vi "Methods to Method Info.vi"(10 "Class":string, 11 "Methods from Node":T2(array[cluster])) -> (2 "Methods for Tree":T1(array[cluster]), 3 "Methods[]":T3(array[cluster]))   [LabVIEW 2023] (continued)
ID string"="22", "Class Name (unlocalized)"="WaveformGraph", "Class Name (localized)"="WaveformGraph"}, "Method Info"={"Unique ID string"="6343003", "Data name"="Export Data to Clipboard", "Short name (localized)"="Export Data to Clipboard", "Long name (localized)"="Export Data to Clipboard"}, "Method Flags"={"IsDeprecated"=FALSE, "IsPrivate"=FALSE, "IsScripting"=FALSE, "IsNotInRun-Time"=FALSE}, "Divider"=FALSE}, {"Class Info"={"Unique ID string"="24", "Parent ID string"="22", "Class Name (unlocalized)"="WaveformGraph", "Class Name (localized)"="WaveformGraph"}, "Method Info"={"Unique ID string"="6343004", "Data name"="Export Data to Excel", "Short name (localized)"="Export Data to Excel", "Long name (localized)"="Export Data to Excel"}, "Method Flags"={"IsDeprecated"=FALSE, "IsPrivate"=FALSE, "IsScripting"=FALSE, "IsNotInRun-Time"=FALSE}, "Divider"=FALSE}, {"Class Info"={"Unique ID string"="24", "Parent ID string"="22", "Class Name (unlocalized)"="WaveformGraph", "Class Name (localized)"="WaveformGraph"}, "Method Info"={"Unique ID string"="6343005", "Data name"="Export Data to DIAdem", "Short name (localized)"="Export Data to DIAdem", "Long name (localized)"="Export Data to DIAdem"}, "Method Flags"={"IsDeprecated"=FALSE, "IsPrivate"=FALSE, "IsScripting"=FALSE, "IsNotInRun-Time"=FALSE}, "Divider"=FALSE}, {"Class Info"={"Unique ID string"="24", "Parent ID string"="22", "Class Name (unlocalized)"="WaveformGraph", "Class Name (localized)"="WaveformGraph"}, "Method Info"={"Unique ID string"="6343006", "Data name"="Export Plot Data To Clipboard", "Short name (localized)"="Export Plot Data To Clipboard", "Long name (localized)"="Export Plot Data To Clipboard"}, "Method Flags"={"IsDeprecated"=FALSE, "IsPrivate"=FALSE, "IsScripting"=FALSE, "IsNotInRun-Time"=FALSE}, "Divider"=FALSE}, {"Class Info"={"Unique ID string"="24", "Parent ID string"="22", "Class Name (unlocalized)"="WaveformGraph", "Class Name (localized)"="WaveformGraph"}, "Method Info"={"Unique ID string"="6343007", "Data name"="Export Plot Data To Excel", "Short name (localized)"="Export Plot Data To Excel", "Long name (localized)"="Export Plot Data To Excel"}, "Method Flags"={"IsDeprecated"=FALSE, "IsPrivate"=FALSE, "IsScripting"=FALSE, "IsNotInRun-Time"=FALSE}, "Divider"=FALSE}, {"Class Info"={"Unique ID string"="24", "Parent ID string"="22", "Class Name (unlocalized)"="WaveformGraph", "Class Name (localized)"="WaveformGraph"}, "Method Info"={"Unique ID string"="6343008", "Data name"="Export Plot Data To DIAdem", "Short name (localized)"="Export Plot Data To DIAdem", "Long name (localized)"="Export Plot Data To DIAdem"}, "Method Flags"={"IsDeprecated"=FALSE, "IsPrivate"=FALSE, "IsScripting"=FALSE, "IsNotInRun-Time"=FALSE}, "Divider"=FALSE}, {"Class Info"={"Unique ID string"="25", "Parent ID string"="22", "Class Name (unlocalized)"="IntensityChart", "Class Name (localized)"="IntensityChart"}, "Method Info"={"Unique ID string"="6343c00", "Data name"="Export Data to Clipboard", "Short name (localized)"="Export Data to Clipboard", "Long name (localized)"="Export Data to Clipboard"}, "Method Flags"={"IsDeprecated"=FALSE, "IsPrivate"=FALSE, "IsScripting"=FALSE, "IsNotInRun-Time"=FALSE}, "Divider"=FALSE}, {"Class Info"={"Unique ID string"="25", "Parent ID string"="22", "Class Name (unlocalized)"="IntensityChart", "Class Name (localized)"="IntensityChart"}, "Method Info"={"Unique ID string"="6343c01", "Data name"="Export Data to Excel", "Short name (localized)"="Export Data to Excel", "Long name (localized)"="Export Data to Excel"}, "Method Flags"={"IsDeprecated"=FALSE, "IsPrivate"=FALSE, "IsScripting"=FALSE, "IsNotInRun-Time"=FALSE}, "Divider"=FALSE}, {"Class Info"={"Unique ID string"="26", "Parent ID string"="22", "Class Name (unlocalized)"="IntensityGraph", "Class Name (localized)"="IntensityGraph"}, "Method Info"={"Unique ID string"="6344800", "Data name"="Export Data to Clipboard", "Short name (localized)"="Export Data to Clipboard", "Long name (localized)"="Export Data to Clipboard"}, "Method Flags"={"IsDeprecated"=FALSE, "IsPrivate"=FALSE, "IsScripting"=FALSE, "IsNotInRun-Time"=FALSE}, "Divider"=FALSE}, {"Class Info"={"Unique ID string"="26", "Parent ID string"="22", "Class Name (unlocalized)"="IntensityGraph", "Class Name (localized)"="IntensityGraph"}, "Method Info"={"Unique ID string"="6344801", "Data name"="Export Data to Excel", "Short name (localized)"="Export Data to Excel", "Long name (localized)"="Export Data to Excel"}, "Method Flags"={"IsDeprecated"=FALSE, "IsPrivate"=FALSE, "IsScripting"=FALSE, "IsNotInRun-Time"=FALSE}, "Divider"=FALSE}, {"Class Info"={"Unique ID string"="27", "Parent ID string"="6", "Class Name (unlocalized)"="String", "Class Name (localized)"="String"}, "Method Info"={"Unique ID string"="6345400", "Data name"="Size to Text", "Short name (localized)"="Size to Text", "Long name (localized)"="Size to Text"}, "Method Flags"={"IsDeprecated"=FALSE, "IsPrivate"=FALSE, "IsScripting"=FALSE, "IsNotInRun-Time"=FALSE}, "Divider"=FALSE}, {"Class Info"={"Unique ID string"="27", "Parent ID string"="6", "Class Name (unlocalized)"="String", "Class Name (localized)"="String"}, "Method Info"={"Unique ID string"="6345401", "Data name"="Get Nth Line", "Short name (localized)"="Get Nth Line", "Long name (localized)"="Get Nth Line"}, "Method Flags"={"IsDeprecated"=FALSE, "IsPrivate"=FALSE, "IsScripting"=FALSE, "IsNotInRun-Time"=FALSE}, "Divider"=FALSE}, {"Class Info"={"Unique ID string"="27", "Parent ID string"="6", "Class Name (unlocalized)"="String", "Class Name (localized)"="String"}, "Method Info"={"Unique ID string"="6345402", "Data name"="ByteOffFromPt", "Short name (localized)"="ByteOffFromPt", "Long name (localized)"="Byte Offset from Point"}, "Method Flags"={"IsDeprecated"=FALSE, "IsPrivate"=FALSE, "IsScripting"=FALSE, "IsNotInRun-Time"=FALSE}, "Divider"=FALSE}, {"Class Info"={"Unique ID string"="27", "Parent ID string"="6", "Class Name (unlocalized)"="String", "Class Name (localized)"="String"}, "Method Info"={"Unique ID string"="6345403", "Data name"="Append String", "Short name (localized)"="Append String", "Long name (localized)"="Append String"}, "Method Flags"={"IsDeprecated"=FALSE, "IsPrivate"=FALSE, "IsScripting"=FALSE, "IsNotInRun-Time"=FALSE}, "Divider"=FALSE}, {"Class Info"={"Unique ID string"="30", "Parent ID string"="6", "Class Name (unlocalized)"="Cluster", "Class Name (localized)"="Cluster"}, "Method Info"={"Unique ID string"="6347800", "Data name"="Set Cluster Order", "Short name (localized)"="Set Cluster Order", "Long name (localized)"="Set Cluster Order"}, "Method Flags"={"IsDeprecated"=FALSE, "IsPrivate"=FALSE, "IsScripting"=TRUE, "IsNotInRun-Time"=FALSE}, "Divider"=FALSE}, {"Class Info"={"Unique ID string"="31", "Parent ID string"="36", "Class Name (unlocalized)"="Panel", "Class Name (localized)"="Panel"}, "Method Info"={"Unique ID string"="6348400", "Data name"="Set Panel Order", "Short name (localized)"="Set Panel Order", "Long name (localized)"="Set Panel Order"}, "Method Flags"={"IsDeprecated"=FALSE, "IsPrivate"=FALSE, "IsScripting"=TRUE, "IsNotInRun-Time"=FALSE}, "Divider"=FALSE}, {"Class Info"={"Unique ID string"="31", "Parent ID string"="36", "Class Name (unlocalized)"="Panel", "Class Name (localized)"="Panel"}, "Method Info"={"Unique ID string"="6348402", "Data name"="Clear Selection", "Short name (localized)"="Clear Selection", "Long name (localized)"="Clear Selection"}, "Method Flags"={"IsDeprecated"=FALSE, "IsPrivate"=FALSE, "IsScripting"=TRUE, "IsNotInRun-Time"=TRUE}, "Divider"=FALSE}, {"Class Info"={"Unique ID string"="31", "Parent ID string"="36", "Class Name (unlocalized)"="Panel", "Class Name (localized)"="Panel"}, "Method Info"={"Unique ID string"="6348403", "Data name"="Make Selection", "Short name (localized)"="Make Selection", "Long name (localized)"="Make Selection"}, "Method Flags"={"IsDeprecated"=FALSE, "IsPrivate"=FALSE, "IsScripting"=TRUE, "IsNotInRun-Time"=TRUE}, "Divider"=FALSE}, {"Class Info"={"Unique ID string"="31", "Parent ID string"="36", "Class Name (unlocalized)"="Panel", "Class Name (localized)"="Panel"}, "Method Info"={"Unique ID string"="6348404", "Data name"="Select All", "Short name (localized)"="Select All", "Long name (localized)"="Select All"}, "Method Flags"={"IsDeprecated"=FALSE, "IsPrivate"=FALSE, "IsScripting"=TRUE, "IsNotInRun-Time"=TRUE}, "Divider"=FALSE}, {"Class Info"={"Unique ID string"="31", "Parent ID string"="36", "Class Name (unlocalized)"="Panel", "Class Name (localized)"="Panel"}, "Method Info"={"Unique ID string"="6348405", "Data name"="Copy Selection", "Short name (localized)"="Copy Selection", "Long name (localized)"="Copy Selection"}, "Method Flags"={"IsDeprecated"=FALSE, "IsPrivate"=FALSE, "IsScripting"=TRUE, "IsNotInRun-Time"=TRUE}, "Divider"=FALSE}, {"Class Info"={"Unique ID string"="31", "Parent ID string"="36", "Class Name (unlocalized)"="Panel", "Class Name (localized)"="Panel"}, "Method Info"={"Unique ID string"="634840b", "Data name"="MoveSelectionToFront", "Short name (localized)"="MoveSelectionToFront", "Long name (localized)"="Move Selection To Front"}, "Method Flags"={"IsDeprecated"=FALSE, "IsPrivate"=FALSE, "IsScripting"=TRUE, "IsNotInRun-Time"=TRUE}, "Divider"=FALSE}, {"Class Info"={"Unique ID string"="31", "Parent ID string"="36", "Class Name (unlocalized)"="Panel", "Class Name (localized)"="Panel"}, "Method Info"={"Unique ID string"="634840c", "Data name"="MoveSelectionToBack", "Short name (localized)"="MoveSelectionToBack", "Long name (localized)"="Move Selection To Back"}, "Method Flags"={"IsDeprecated"=FALSE, "IsPrivate"=FALSE, "IsScripting"=TRUE, "IsNotInRun-Time"=TRUE}, "Divider"=FALSE}, {"Class Info"={"Unique ID string"="31", "Parent ID string"="36", "Class Name (unlocalized)"="Panel", "Class Name (localized)"="Panel"}, "Method Info"={"Unique ID string"="634840d", "Data name"="MoveSelectionForward", "Short name (localized)"="MoveSelectionForward", "Long name (localized)"="Move Selection Forward"}, "Method Flags"={"IsDeprecated"=FALSE, "IsPrivate"=FALSE, "IsScripting"=TRUE, "IsNotInRun-Time"=TRUE}, "Divider"=FALSE}, {"Class Info"={"Unique ID string"="31", "Parent ID string"="36", "Class Name (unlocalized)"="Panel", "Class Name (localized)"="Panel"}, "Method Info"={"Unique ID string"="634840e", "Data name"="MoveSelectionBackward", "Short name (localized)"="MoveSelectionBackward", "Long name (localized)"="Move Selection Backward"}, "Method Flags"={"IsDeprecated"=FALSE, "IsPrivate"=FALSE, "IsScripting"=TRUE, "IsNotInRun-Time"=TRUE}, "Divider"=FALSE}, {"Class Info"={"Unique ID string"="31", "Parent ID string"="36", "Class Name (unlocalized)"="Panel", "Class Name (localized)"="Panel"}, "Method Info"={"Unique ID string"="634840f", "Data name"="CvtPanelToScreenCoords", "Short name (localized)"="CvtPanelToScreenCoords", "Long name (localized)"="Convert Panel To Screen Coordinates"}, "Method Flags"={"IsDeprecated"=FALSE, "IsPrivate"=FALSE, "IsScripting"=FALSE, "IsNotInRun-Time"=FALSE}, "Divider"=FALSE}, {"Class Info"={"Unique ID string"="31", "Parent ID string"="36", "Class Name (unlocalized)"="Panel", "Class Name (localized)"="Panel"}, "Method Info"={"Unique ID string"="6348410", "Data name"="CvtScreenToPanelCoords", "Short name (localized)"="CvtScreenToPanelCoords", "Long name (localized)"="Convert Screen To Panel Coordinates"}, "Method Flags"={"IsDeprecated"=FALSE, "IsPrivate"=FALSE, "IsScripting"=FALSE, "IsNotInRun-Time"=FALSE}, "Divider"=FALSE}, {"Class Info"={"Unique ID string"="31", "Parent ID string"="36", "Class Name (unlocalized)"="Panel", "Class Name (localized)"="Panel"}, "Method Info"={"Unique ID string"="6348411", "Data name"="DistributeSelection", "Short name (localized)"="DistributeSelection", "Long name (localized)"="Distribute Selection"}, "Method Flags"={"IsDeprecated"=FALSE, "IsPrivate"=FALSE, "IsScripting"=TRUE, "IsNotInRun-Time"=TRUE}, "Divider"=FALSE}, {"Class Info"={"Unique ID string"="31", "Parent ID string"="36", "Class Name (unlocalized)"="Panel", "Class Name (localized)"="Panel"}, "Method Info"={"Unique ID string"="6348412", "Data name"="AlignSelection", "Short name (localized)"="AlignSelection", "Long name (localized)"="Align Selection"}, "Method Flags"={"IsDeprecated"=FALSE, "IsPrivate"=FALSE, "IsScripting"=TRUE, "IsNotInRun-Time"=TRUE}, "Divider"=FALSE}, {"Class Info"={"Unique ID string"="33", "Parent ID string"="17", "Class Name (unlocalized)"="NumericWithScale", "Class Name (localized)"="NumericWithScale"}, "Method Info"={"Unique ID string"="633f400", "Data name"="Add Slider", "Short name (localized)"="Add Slider", "Long name (localized)"="Add Slider"}, "Method Flags"={"IsDeprecated"=FALSE, "IsPrivate"=FALSE, "IsScripting"=TRUE, "IsNotInRun-Time"=TRUE}, "Divider"=FALSE}, {"Class Info"={"Unique ID string"="33", "Parent ID string"="17", "Class Name (unlocalized)"="NumericWithScale", "Class Name (localized)"="NumericWithScale"}, "Method Info"={"Unique ID string"="633f401", "Data name"="Delete Slider", "Short name (localized)"="Delete Slider", "Long name (localized)"="Delete Slider"}, "Method Flags"={"IsDeprecated"=FALSE, "IsPrivate"=FALSE, "IsScripting"=TRUE, "IsNotInRun-Time"=TRUE}, "Divider"=FALSE}, {"Class Info"={"Unique ID string"="36", "Parent ID string"="3", "Class Name (unlocalized)"="GObject", "Class Name (localized)"="GObject"}, "Method Info"={"Unique ID string"="632a400", "Data name"="Move", "Short name (localized)"="Move", "Long name (localized)"="Move"}, "Method Flags"={"IsDeprecated"=FALSE, "IsPrivate"=FALSE, "IsScripting"=TRUE, "IsNotInRun-Time"=TRUE}, "Divider"=FALSE}, {"Class Info"={"Unique ID string"="36", "Parent ID string"="3", "Class Name (unlocalized)"="GObject", "Class Name (localized)"="GObject"}, "Method Info"={"Unique ID string"="632a401", "Data name"="ObjHighlight", "Short name (localized)"="ObjHighlight", "Long name (localized)"="Object Highlight"}, "Method Flags"={"IsDeprecated"=FALSE, "IsPrivate"=FALSE, "IsScripting"=FALSE, "IsNotInRun-Time"=FALSE}, "Divider"=FALSE}, {"Class Info"={"Unique ID string"="36", "Parent ID string"="3", "Class Name (unlocalized)"="GObject", "Class Name (localized)"="GObject"}, "Method Info"={"Unique ID string"="632a402", "Data name"="Replace", "Short name (localized)"="Replace", "Long name (localized)"="Replace"}, "Method Flags"={"IsDeprecated"=FALSE, "IsPrivate"=FALSE, "IsScripting"=TRUE, "IsNotInRun-Time"=TRUE}, "Divider"=FALSE}, {"Class Info"={"Unique ID string"="36", "Parent ID string"="3", "Class Name (unlocalized)"="GObject", "Class Name (localized)"="GObject"}, "Method Info"={"Unique ID string"="632a403", "Data name"="Replace No Attrib", "Short name (localized)"="Replace No Attrib", "Long name (localized)"="Replace No Attributes"}, "Method Flags"={"IsDeprecated"=FALSE, "IsPrivate"=FALSE, "IsScripting"=TRUE, "IsNotInRun-Time"=TRUE}, "Divider"=FALSE}, {"Class Info"={"Unique ID string"="36", "Parent ID string"="3", "Class Name (unlocalized)"="GObject", "Class Name (localized)"="GObject"}, "Method Info"={"Unique ID string"="632a404", "Data name"="Launch Config", "Short name (localized)"="Launch Config", "Long name (localized)"="Launch Config Page"}, "Method Flags"={"IsDeprecated"=FALSE, "IsPrivate"=TRUE, "IsScripting"=TRUE, "IsNotInRun-Time"=TRUE}, "Divider"=FALSE}, {"Class Info"={"Unique ID string"="36", "Parent ID string"="3", "Class Name (unlocalized)"="GObject", "Class Name (localized)"="GObject"}, "Method Info"={"Unique ID string"="632a405", "Data name"="Invalidate", "Short name (localized)"="Invalidate", "Long name (localized)"="Invalidate"}, "Method Flags"={"IsDeprecated"=FALSE, "IsPrivate"=TRUE, "IsScripting"=TRUE, "IsNotInRun-Time"=FALSE}, "Divider"=FALSE}, {"Class Info"={"Unique ID string"="36", "Parent ID string"="3", "Class Name (unlocalized)"="GObject", "Class Name (localized)"="GObject"}, "Method Info"={"Unique ID string"="632a406", "Data name"="ReplacePreferringStubDDOOnFP", "Short name (localized)"="ReplacePreferringStubDDOOnFP", "Long name (localized)"="Replace Preferring Stub DDO OnFP"}, "Method Flags"={"IsDeprecated"=FALSE, "IsPrivate"=TRUE, "IsScripting"=TRUE, "IsNotInRun-Time"=TRUE}, "Divider"=FALSE}, {"Class Info"={"Unique ID string"="36", "Parent ID string"="3", "Class Name (unlocalized)"="GObject", "Class Name (localized)"="GObject"}, "Method Info"={"Unique ID string"="632a407", "Data name"="GetObjHelp", "Short name (localized)"="GetObjHelp", "Long name (localized)"="Get Help Info"}, "Method Flags"={"IsDeprecated"=FALSE, "IsPrivate"=FALSE, "IsScripting"=TRUE, "IsNotInRun-Time"=FALSE}, "Divider"=FALSE}, {"Class Info"={"Unique ID string"="46", "Parent ID string"="6", "Class Name (unlocalized)"="MulticolumnListbox", "Class Name (localized)"="MulticolumnListbox"}, "Method Info"={"Unique ID string"="18d99400", "Data name"="Get DblClk Row", "Short name (localized)"="Get DblClk Row", "Long name (localized)"="Get Double-Clicked Row"}, "Method Flags"={"IsDeprecated"=FALSE, "IsPrivate"=FALSE, "IsScripting"=FALSE, "IsNotInRun-Time"=FALSE}, "Divider"=FALSE}, {"Class Info"={"Unique ID string"="46", "Parent ID string"="6", "Class Name (unlocalized)"="MulticolumnListbox", "Class Name (localized)"="MulticolumnListbox"}, "Method Info"={"Unique ID string"="18d99401", "Data name"="Get Clicked Col Hdr", "Short name (localized)"="Get Clicked Col Hdr", "Long name (localized)"="Get Clicked Column Header"}, "Method Flags"={"IsDeprecated"=FALSE, "IsPrivate"=FALSE, "IsScripting"=FALSE, "IsNotInRun-Time"=FALSE}, "Divider"=FALSE}, {"Class Info"={"Unique ID string"="46", "Parent ID string"="6", "Class Name (unlocalized)"="MulticolumnListbox", "Class Name (localized)"="MulticolumnListbox"}, "Method Info"={"Unique ID string"="18d99402", "Data name"="Point To Row Column", "Short name (localized)"="Point To Row Column", "Long name (localized)"="Point to Row Column"}, "Method Flags"={"IsDeprecated"=FALSE, "IsPrivate"=FALSE, "IsScripting"=FALSE, "IsNotInRun-Time"=FALSE}, "Divider"=FALSE}, {"Class Info"={"Unique ID string"="46", "Parent ID string"="6", "Class Name (unlocalized)"="MulticolumnListbox", "Class Name (localized)"="MulticolumnListbox"}, "Method Info"={"Unique ID string"="18d99403", "Data name"="Custom Item Symbols.Get Symbol", "Short name (localized)"="Custom Item Symbols.Get Symbol", "Long name (localized)"="Custom Item Symbols:Get Symbol"}, "Method Flags"={"IsDeprecated"=FALSE, "IsPrivate"=FALSE, "IsScripting"=FALSE, "IsNotInRun-Time"=FALSE}, "Divider"=FALSE}, {"Class Info"={"Unique ID string"="46", "Parent ID string"="6", "Class Name (unlocalized)"="MulticolumnListbox", "Class Name (localized)"="MulticolumnListbox"}, "Method Info"={"Unique ID string"="18d99404", "Data name"="Custom Item Symbols.Get Symbol Array", "Short name (localized)"="Custom Item Symbols.Get Symbol Array", "Long name (localized)"="Custom Item Symbols:Get Symbol Array"}, "Method Flags"={"IsDeprecated"=FALSE, "IsPrivate"=FALSE, "IsScripting"=FALSE, "IsNotInRun-Time"=FALSE}, "Divider"=FALSE}, {"Class Info"={"Unique ID string"="46", "Parent ID string"="6", "Class Name (unlocalized)"="MulticolumnListbox", "Class Name (localized)"="MulticolumnListbox"}, "Method Info"={"Unique ID string"="18d99405", "Data name"="Custom Item Symbols.Set Symbol", "Short name (localized)"="Custom Item Symbols.Set Symbol", "Long name (localized)"="Custom Item Symbols:Set To Custom Symbol"}, "Method Flags"={"IsDeprecated"=FALSE, "IsPrivate"=FALSE, "IsScripting"=FALSE, "IsNotInRun-Time"=FALSE}, "Divider"=FALSE}, {"Class Info"={"Unique ID string"="46", "Parent ID string"="6", "Class Name (unlocalized)"="MulticolumnListbox", "Class Name (localized)"="MulticolumnListbox"}, "Method Info"={"Unique ID string"="18d99406", "Data name"="Custom Item Symbols.Set Symbol Array", "Short name (localized)"="Custom Item Symbols.Set Symbol Array", "Long name (localized)"="Custom Item Symbols:Set To Custom Symbol Array"}, "Method Flags"={"IsDeprecated"=FALSE, "IsPrivate"=FALSE, "IsScripting"=FALSE, "IsNotInRun-Time"=FALSE}, "Divider"=FALSE}, {"Class Info"={"Unique ID string"="46", "Parent ID string"="6", "Class Name (unlocalized)"="MulticolumnListbox", "Class Name (localized)"="MulticolumnListbox"}, "Method Info"={"Unique ID string"="18d99407", "Data name"="Custom Item Symbols.Revert Symbol", "Short name (localized)"="Custom Item Symbols.Revert Symbol", "Long name (localized)"="Custom Item Symbols:Revert To Built In Symbol"}, "Method Flags"={"IsDeprecated"=FALSE, "IsPrivate"=FALSE, "IsScripting"=FALSE, "IsNotInRun-Time"=FALSE}, "Divider"=FALSE}, {"Class Info"={"Unique ID string"="46", "Parent ID string"="6", "Class Name (unlocalized)"="MulticolumnListbox", "Class Name (localized)"="MulticolumnListbox"}, "Method Info"={"Unique ID string"="18d99408", "Data name"="Custom Item Symbols.Revert Symbols", "Short name (localized)"="Custom Item Symbols.Revert Symbols", "Long name (localized)"="Custom Item Symbols:Revert All To Built In Symbols"}, "Method Flags"={"IsDeprecated"=FALSE, "IsPrivate"=FALSE, "IsScripting"=FALSE, "IsNotInRun-Time"=FALSE}, "Divider"=FALSE}, {"Class Info"={"Unique ID string"="50", "Parent ID string"="28", "Class Name (unlocalized)"="VISAResourceName", "Class Name (localized)"="VISAResourceName"}, "Method Info"={"Unique ID string"="6354b000", "Data name"="SetClassName", "Short name (localized)"="SetClassName", "Long name (localized)"="Set Class Name"}, "Method Flags"={"IsDeprecated"=FALSE, "IsPrivate"=TRUE, "IsScripting"=FALSE, "IsNotInRun-Time"=FALSE}, "Divider"=FALSE}, {"Class Info"={"Unique ID string"="51", "Parent ID string"="28", "Class Name (unlocalized)"="IVILogicalName", "Class Name (localized)"="IVILogicalName"}, "Method Info"={"Unique ID string"="667cb800", "Data name"="SetClassName", "Short name (localized)"="SetClassName", "Long name (localized)"="Set Class Name"}, "Method Flags"={"IsDeprecated"=FALSE, "IsPrivate"=TRUE, "IsScripting"=FALSE, "IsNotInRun-Time"=FALSE}, "Divider"=FALSE}, {"Class Info"={"Unique ID string"="53", "Parent ID string"="6", "Class Name (unlocalized)"="PageSelector", "Class Name (localized)"="PageSelector"}, "Method Info"={"Unique ID string"="3e90c00", "Data name"="Remove Page", "Short name (localized)"="Remove Page", "Long name (localized)"="Remove Page"}, "Method Flags"={"IsDeprecated"=FALSE, "IsPrivate"=FALSE, "IsScripting"=TRUE, "IsNotInRun-Time"=TRUE}, "Divider"=FALSE}, {"Class Info"={"Unique ID string"="53", "Parent ID string"="6", "Class Name (unlocalized)"="PageSelector", "Class Name (localized)"="PageSelector"}, "Method Info"={"Unique ID string"="3e90c01", "Data name"="Add Page", "Short name (localized)"="Add Page", "Long name (localized)"="Add Page"}, "Method Flags"={"IsDeprecated"=FALSE, "IsPrivate"=FALSE, "IsScripting"=TRUE, "IsNotInRun-Time"=TRUE}, "Divider"=FALSE}, {"Class Info"={"Unique ID string"="53", "Parent ID string"="6", "Class Name (unlocalized)"="PageSelector", "Class Name (localized)"="PageSelector"}, "Method Info"={"Unique ID string"="3e90c02", "Data name"="Dup Page", "Short name (localized)"="Dup Page", "Long name (localized)"="Duplicate Page"}, "Method Flags"={"IsDeprecated"=FALSE, "IsPrivate"=FALSE, "IsScripting"=TRUE, "IsNotInRun-Time"=TRUE}, "Divider"=FALSE}, {"Class Info"={"Unique ID string"="54", "Parent ID string"="3", "Class Name (unlocalized)"="Page", "Class Name (localized)"="Page"}, "Method Info"={"Unique ID string"="18044800", "Data name"="Reorder Controls", "Short name (localized)"="Reorder Controls", "Long name (localized)"="Reorder Controls"}, "Method Flags"={"IsDeprecated"=FALSE, "IsPrivate"=FALSE, "IsScripting"=TRUE, "IsNotInRun-Time"=FALSE}, "Divider"=FALSE}, {"Class Info"={"Unique ID string"="54", "Parent ID string"="3", "Class Name (unlocalized)"="Page", "Class Name (localized)"="Page"}, "Method Info"={"Unique ID string"="18044801", "Data name"="Import Image", "Short name (localized)"="Import Image", "Long name (localized)"="Import Image"}, "Method Flags"={"IsDeprecated"=FALSE, "IsPrivate"=FALSE, "IsScripting"=FALSE, "IsNotInRun-Time"=FALSE}, "Divider"=FALSE}, {"Class Info"={"Unique ID string"="54", "Parent ID string"="3", "Class Name (unlocalized)"="Page", "Class Name (localized)"="Page"}, "Method Info"={"Unique ID string"="18044802", "Data name"="Remove Image", "Short name (localized)"="Remove Image", "Long name (localized)"="Remove Image"}, "Method Flags"={"IsDeprecated"=FALSE, "IsPrivate"=FALSE, "IsScripting"=FALSE, "IsNotInRun-Time"=FALSE}, "Divider"=FALSE}, {"Class Info"={"Unique ID string"="55", "Parent ID string"="53", "Class Name (unlocalized)"="TabControl", "Class Name (localized)"="TabControl"}, "Method Info"={"Unique ID string"="24deb000", "Data name"="Rearrange Pages", "Short name (localized)"="Rearrange Pages", "Long name (localized)"="Rearrange Pages"}, "Method Flags"={"IsDeprecated"=FALSE, "IsPrivate"=FALSE, "IsScripting"=TRUE, "IsNotInRun-Time"=FALSE}, "Divider"=FALSE}, {"Class Info"={"Unique ID string"="56", "Parent ID string"="3", "Class Name (unlocalized)"="ConnectorPane", "Class Name (localized)"="ConnectorPane"}, "Method Info"={"Unique ID string"="239a8000", "Data name"="AssignCtrlToTerm", "Short name (localized)"="AssignCtrlToTerm", "Long name (localized)"="Assign Control To Terminal"}, "Method Flags"={"IsDeprecated"=FALSE, "IsPrivate"=FALSE, "IsScripting"=TRUE, "IsNotInRun-Time"=TRUE}, "Divider"=FALSE}, {"Class Info"={"Unique ID string"="56", "Parent ID string"="3", "Class Name (unlocalized)"="ConnectorPane", "Class Name (localized)"="ConnectorPane"}, "Method Info"={"Unique ID string"="239a8001", "Data name"="SetWireRule", "Short name (localized)"="SetWireRule", "Long name (localized)"="Wiring Rule:Set"}, "Method Flags"={"IsDeprecated"=FALSE, "IsPrivate"=FALSE, "IsScripting"=TRUE, "IsNotInRun-Time"=TRUE}, "Divider"=FALSE}, {"Class Info"={"Unique ID string"="56", "Parent ID string"="3", "Class Name (unlocalized)"="ConnectorPane", "Class Name (localized)"="ConnectorPane"}, "Method Info"={"Unique ID string"="239a8002", "Data name"="DiscTerm", "Short name (localized)"="DiscTerm", "Long name (localized)"="Disconnect Terminal"}, "Method Flags"={"IsDeprecated"=FALSE, "IsPrivate"=FALSE, "IsScripting"=TRUE, "IsNotInRun-Time"=TRUE}, "Divider"=FALSE}, {"Class Info"={"Unique ID string"="56", "Parent ID string"="3", "Class Name (unlocalized)"="ConnectorPane", "Class Name (localized)"="ConnectorPane"}, "Method Info"={"Unique ID string"="239a8003", "Data name"="DiscAllTerms", "Short name (localized)"="DiscAllTerms", "Long name (localized)"="Disconnect All Terminals"}, "Method Flags"={"IsDeprecated"=FALSE, "IsPrivate"=FALSE, "IsScripting"=TRUE, "IsNotInRun-Time"=TRUE}, "Divider"=FALSE}, {"Class Info"={"Unique ID string"="56", "Parent ID string"="3", "Class Name (unlocalized)"="ConnectorPane", "Class Name (localized)"="ConnectorPane"}, "Method Info"={"Unique ID string"="239a8004", "Data name"="Rot90", "Short name (localized)"="Rot90", "Long name (localized)"="Rotate By 90"}, "Method Flags"={"IsDeprecated"=FALSE, "IsPrivate"=FALSE, "IsScripting"=TRUE, "IsNotInRun-Time"=TRUE}, "Divider"=FALSE}, {"Class Info"={"Unique ID string"="56", "Parent ID string"="3", "Class Name (unlocalized)"="ConnectorPane", "Class Name (localized)"="ConnectorPane"}, "Method Info"={"Unique ID string"="239a8005", "Data name"="FlipHoriz", "Short name (localized)"="FlipHoriz", "Long name (localized)"="Flip Horizontal"}, "Method Flags"={"IsDeprecated"=FALSE, "IsPrivate"=FALSE, "IsScripting"=TRUE, "IsNotInRun-Time"=TRUE}, "Divider"=FALSE}, {"Class Info"={"Unique ID string"="56", "Parent ID string"="3", "Class Name (unlocalized)"="ConnectorPane", "Class Name (localized)"="ConnectorPane"}, "Method Info"={"Unique ID string"="239a8006", "Data name"="FlipVert", "Short name (localized)"="FlipVert", "Long name (localized)"="Flip Vertical"}, "Method Flags"={"IsDeprecated"=FALSE, "IsPrivate"=FALSE, "IsScripting"=TRUE, "IsNotInRun-Time"=TRUE}, "Divider"=FALSE}, {"Class Info"={"Unique ID string"="56", "Parent ID string"="3", "Class Name (unlocalized)"="ConnectorPane", "Class Name (localized)"="ConnectorPane"}, "Method Info"={"Unique ID string"="239a8007", "Data name"="GetWiringRule", "Short name (localized)"="GetWiringRule", "Long name (localized)"="Wiring Rule:Get"}, "Method Flags"={"IsDeprecated"=FALSE, "IsPrivate"=FALSE, "IsScripting"=TRUE, "IsNotInRun-Time"=TRUE}, "Divider"=FALSE}, {"Class Info"={"Unique ID string"="58", "Parent ID string"="59", "Class Name (unlocalized)"="VIRefNum", "Class Name (localized)"="VIRefNum"}, "Method Info"={"Unique ID string"="699be000", "Data name"="Make Strict Reference", "Short name (localized)"="Make Strict Reference", "Long name (localized)"="Make Strict Reference"}, "Method Flags"={"IsDeprecated"=FALSE, "IsPrivate"=FALSE, "IsScripting"=TRUE, "IsNotInRun-Time"=FALSE}, "Divider"=FALSE}, {"Class Info"={"Unique ID string"="58", "Parent ID string"="59", "Class Name (unlocalized)"="VIRefNum", "Class Name (localized)"="VIRefNum"}, "Method Info"={"Unique ID string"="699be001", "Data name"="Make Non-Strict Reference", "Short name (localized)"="Make Non-Strict Reference", "Long name (localized)"="Make Non-Strict Reference"}, "Method Flags"={"IsDeprecated"=FALSE, "IsPrivate"=FALSE, "IsScripting"=TRUE, "IsNotInRun-Time"=FALSE}, "Divider"=FALSE}, {"Class Info"={"Unique ID string"="58", "Parent ID string"="59", "Class Name (unlocalized)"="VIRefNum", "Class Name (localized)"="VIRefNum"}, "Method Info"={"Unique ID string"="699be003", "Data name"="Set Conpane", "Short name (localized)"="Set Conpane", "Long name (localized)"="Set Conpane"}, "Method Flags"={"IsDeprecated"=FALSE, "IsPrivate"=FALSE, "IsScripting"=TRUE, "IsNotInRun-Time"=TRUE}, "Divider"=FALSE}, {"Class Info"={"Unique ID string"="61", "Parent ID string"="6", "Class Name (unlocalized)"="DigitalTable", "Class Name (localized)"="DigitalTable"}, "Method Info"={"Unique ID string"="7494bc00", "Data name"="Point To Row Column", "Short name (localized)"="Point To Row Column", "Long name (localized)"="Point to Row Column"}, "Method Flags"={"IsDeprecated"=FALSE, "IsPrivate"=FALSE, "IsScripting"=FALSE, "IsNotInRun-Time"=FALSE}, "Divider"=FALSE}, {"Class Info"={"Unique ID string"="61", "Parent ID string"="6", "Class Name (unlocalized)"="DigitalTable", "Class Name (localized)"="DigitalTable"}, "Method Info"={"Unique ID string"="7494bc01", "Data name"="ExportImage", "Short name (localized)"="ExportImage", "Long name (localized)"="Export Image"}, "Method Flags"={"IsDeprecated"=FALSE, "IsPrivate"=FALSE, "IsScripting"=FALSE, "IsNotInRun-Time"=FALSE}, "Divider"=FALSE}, {"Class Info"={"Unique ID string"="61", "Parent ID string"="6", "Class Name (unlocalized)"="DigitalTable", "Class Name (localized)"="DigitalTable"}, "Method Info"={"Unique ID string"="7494bc02", "Data name"="ExportImage Color", "Short name (localized)"="ExportImage Color", "Long name (localized)"="Export Image Color"}, "Method Flags"={"IsDeprecated"=FALSE, "IsPrivate"=TRUE, "IsScripting"=FALSE, "IsNotInRun-Time"=FALSE}, "Divider"=FALSE}, {"Class Info"={"Unique ID string"="61", "Parent ID string"="6", "Class Name (unlocalized)"="DigitalTable", "Class Name (localized)"="DigitalTable"}, "Method Info"={"Unique ID string"="7494bc03", "Data name"="Export Data to Clipboard", "Short name (localized)"="Export Data to Clipboard", "Long name (localized)"="Export Data to Clipboard"}, "Method Flags"={"IsDeprecated"=FALSE, "IsPrivate"=FALSE, "IsScripting"=FALSE, "IsNotInRun-Time"=FALSE}, "Divider"=FALSE}, {"Class Info"={"Unique ID string"="61", "Parent ID string"="6", "Class Name (unlocalized)"="DigitalTable", "Class Name (localized)"="DigitalTable"}, "Method Info"={"Unique ID string"="7494bc04", "Data name"="Export Data to Excel", "Short name (localized)"="Export Data to Excel", "Long name (localized)"="Export Data to Excel"}, "Method Flags"={"IsDeprecated"=FALSE, "IsPrivate"=FALSE, "IsScripting"=FALSE, "IsNotInRun-Time"=FALSE}, "Divider"=FALSE}, {"Class Info"={"Unique ID string"="65", "Parent ID string"="6", "Class Name (unlocalized)"="SubPanel", "Class Name (localized)"="SubPanel"}, "Method Info"={"Unique ID string"="72583c00", "Data name"="Insert VI", "Short name (localized)"="Insert VI", "Long name (localized)"="Insert VI"}, "Method Flags"={"IsDeprecated"=FALSE, "IsPrivate"=FALSE, "IsScripting"=FALSE, "IsNotInRun-Time"=FALSE}, "Divider"=FALSE}, {"Class Info"={"Unique ID string"="65", "Parent ID string"="6", "Class Name (unlocalized)"="SubPanel", "Class Name (localized)"="SubPanel"}, "Method Info"={"Unique ID string"="72583c01", "Data name"="Remove VI", "Short name (localized)"="Remove VI", "Long name (localized)"="Remove VI"}, "Method Flags"={"IsDeprecated"=FALSE, "IsPrivate"=FALSE, "IsScripting"=FALSE, "IsNotInRun-Time"=FALSE}, "Divider"=FALSE}, {"Class Info"={"Unique ID string"="65", "Parent ID string"="6", "Class Name (unlocalized)"="SubPanel", "Class Name (localized)"="SubPanel"}, "Method Info"={"Unique ID string"="72583c02", "Data name"="InsertBD", "Short name (localized)"="InsertBD", "Long name (localized)"="InsertBlockDiagram"}, "Method Flags"={"IsDeprecated"=FALSE, "IsPrivate"=FALSE, "IsScripting"=TRUE, "IsNotInRun-Time"=FALSE}, "Divider"=FALSE}, {"Class Info"={"Unique ID string"="65", "Parent ID string"="6", "Class Name (unlocalized)"="SubPanel", "Class Name (localized)"="SubPanel"}, "Method Info"={"Unique ID string"="72583c03", "Data name"="Insert Remote VI", "Short name (localized)"="Insert Remote VI", "Long name (localized)"="Insert Remote VI"}, "Method Flags"={"IsDeprecated"=FALSE, "IsPrivate"=TRUE, "IsScripting"=FALSE, "IsNotInRun-Time"=FALSE}, "Divider"=FALSE}, {"Class Info"={"Unique ID string"="66", "Parent ID string"="6", "Class Name (unlocalized)"="TreeControl", "Class Name (localized)"="TreeControl"}, "Method Info"={"Unique ID string"="756a3800", "Data name"="Navigate Tree.Get Next", "Short name (localized)"="Navigate Tree.Get Next", "Long name (localized)"="Navigate Tree:Get Next Item"}, "Method Flags"={"IsDeprecated"=FALSE, "IsPrivate"=FALSE, "IsScripting"=FALSE, "IsNotInRun-Time"=FALSE}, "Divider"=FALSE}, {"Class Info"={"Unique ID string"="66", "Parent ID string"="6", "Class Name (unlocalized)"="TreeControl", "Class Name (localized)"="TreeControl"}, "Method Info"={"Unique ID string"="756a3801", "Data name"="Navigate Tree.Get Parent", "Short name (localized)"="Navigate Tree.Get Parent", "Long name (localized)"="Navigate Tree:Get Parent Item"}, "Method Flags"={"IsDeprecated"=FALSE, "IsPrivate"=FALSE, "IsScripting"=FALSE, "IsNotInRun-Time"=FALSE}, "Divider"=FALSE}, {"Class Info"={"Unique ID string"="66", "Parent ID string"="6", "Class Name (unlocalized)"="TreeControl", "Class Name (localized)"="TreeControl"}, "Method Info"={"Unique ID string"="756a3802", "Data name"="Navigate Tree.Get Path", "Short name (localized)"="Navigate Tree.Get Path", "Long name (localized)"="Navigate Tree:Get Path"}, "Method Flags"={"IsDeprecated"=FALSE, "IsPrivate"=FALSE, "IsScripting"=FALSE, "IsNotInRun-Time"=FALSE}, "Divider"=FALSE}, {"Class Info"={"Unique ID string"="66", "Parent ID string"="6", "Class Name (unlocalized)"="TreeControl", "Class Name (localized)"="TreeControl"}, "Method Info"={"Unique ID string"="756a3803", "Data name"="Edit Tree Items.Delete", "Short name (localized)"="Edit Tree Items.Delete", "Long name (localized)"="Edit Tree Items:Delete Item"}, "Method Flags"={"IsDeprecated"=FALSE, "IsPrivate"=FALSE, "IsScripting"=FALSE, "IsNotInRun-Time"=FALSE}, "Divider"=FALSE}, {"Class Info"={"Unique ID string"="66", "Parent ID string"="6", "Class Name (unlocalized)"="TreeControl", "Class Name (localized)"="TreeControl"}, "Method Info"={"Unique ID string"="756a3804", "Data name"="Edit Tree Items.Add Item", "Short name (localized)"="Edit Tree Items.Add Item", "Long name (localized)"="Edit Tree Items:Add Item"}, "Method Flags"={"IsDeprecated"=FALSE, "IsPrivate"=FALSE, "IsScripting"=FALSE, "IsNotInRun-Time"=FALSE}, "Divider"=FALSE}, {"Class Info"={"Unique ID string"="66", "Parent ID string"="6", "Class Name (unlocalized)"="TreeControl", "Class Name (localized)"="TreeControl"}, "Method Info"={"Unique ID string"="756a3805", "Data name"="Edit Tree Items.Add Item to End", "Short name (localized)"="Edit Tree Items.Add Item to End", "Long name (localized)"="Edit Tree Items:Add Item to End"}, "Method Flags"={"IsDeprecated"=FALSE, "IsPrivate"=FALSE, "IsScripting"=FALSE, "IsNotInRun-Time"=FALSE}, "Divider"=FALSE}, {"Class Info"={"Unique ID string"="66", "Parent ID string"="6", "Class Name (unlocalized)"="TreeControl", "Class Name (localized)"="TreeControl"}, "Method Info"={"Unique ID string"="756a3806", "Data name"="Open/Close.Item", "Short name (localized)"="Open/Close.Item", "Long name (localized)"="Open/Close:Item"}, "Method Flags"={"IsDeprecated"=FALSE, "IsPrivate"=FALSE, "IsScripting"=FALSE, "IsNotInRun-Time"=FALSE}, "Divider"=FALSE}, {"Class Info"={"Unique ID string"="66", "Parent ID string"="6", "Class Name (unlocalized)"="TreeControl", "Class Name (localized)"="TreeControl"}, "Method Info"={"Unique ID string"="756a3807", "Data name"="Edit Tree Items.Sort Children", "Short name (localized)"="Edit Tree Items.Sort Children", "Long name (localized)"="Edit Tree Items:Sort Children"}, "Method Flags"={"IsDeprecated"=FALSE, "IsPrivate"=FALSE, "IsScripting"=FALSE, "IsNotInRun-Time"=FALSE}, "Divider"=FALSE}, {"Class Info"={"Unique ID string"="66", "Parent ID string"="6", "Class Name (unlocalized)"="TreeControl", "Class Name (localized)"="TreeControl"}, "Method Info"={"Unique ID string"="756a3808", "Data name"="Open/Close.Ensure Visible", "Short name (localized)"="Open/Close.Ensure Visible", "Long name (localized)"="Open/Close:Ensure Visible"}, "Method Flags"={"IsDeprecated"=FALSE, "IsPrivate"=FALSE, "IsScripting"=FALSE, "IsNotInRun-Time"=FALSE}, "Divider"=FALSE}, {"Class Info"={"Unique ID string"="66", "Parent ID string"="6", "Class Name (unlocalized)"="TreeControl", "Class Name (localized)"="TreeControl"}, "Method Info"={"Unique ID string"="756a3809", "Data name"="Open/Close.Open/Close All", "Short name (localized)"="Open/Close.Open/Close All", "Long name (localized)"="Open/Close:All"}, "Method Flags"={"IsDeprecated"=FALSE, "IsPrivate"=FALSE, "IsScripting"=FALSE, "IsNotInRun-Time"=FALSE}, "Divider"=FALSE}, {"Class Info"={"Unique ID string"="66", "Parent ID string"="6", "Class Name (unlocalized)"="TreeControl", "Class Name (localized)"="TreeControl"}, "Method Info"={"Unique ID string"="756a380a", "Data name"="Double Click", "Short name (localized)"="Double Click", "Long name (localized)"="Double Click"}, "Method Flags"={"IsDeprecated"=FALSE, "IsPrivate"=FALSE, "IsScripting"=FALSE, "IsNotInRun-Time"=FALSE}, "Divider"=FALSE}, {"Class Info"={"Unique ID string"="66", "Parent ID string"="6", "Class Name (unlocalized)"="TreeControl", "Class Name (localized)"="TreeControl"}, "Method Info"={"Unique ID string"="756a380c", "Data name"="Edit Tree Items.Move Item", "Short name (localized)"="Edit Tree Items.Move Item", "Long name (localized)"="Edit Tree Items:Move Item"}, "Method Flags"={"IsDeprecated"=FALSE, "IsPrivate"=FALSE, "IsScripting"=FALSE, "IsNotInRun-Time"=FALSE}, "Divider"=FALSE}, {"Class Info"={"Unique ID string"="66", "Parent ID string"="6", "Class Name (unlocalized)"="TreeControl", "Class Name (localized)"="TreeControl"}, "Method Info"={"Unique ID string"="756a380d", "Data name"="Navigate Tree.Get Child", "Short name (localized)"="Navigate Tree.Get Child", "Long name (localized)"="Navigate Tree:Get Child"}, "Method Flags"={"IsDeprecated"=FALSE, "IsPrivate"=FALSE, "IsScripting"=FALSE, "IsNotInRun-Time"=FALSE}, "Divider"=FALSE}, {"Class Info"={"Unique ID string"="66", "Parent ID string"="6", "Class Name (unlocalized)"="TreeControl", "Class Name (localized)"="TreeControl"}, "Method Info"={"Unique ID string"="756a380e", "Data name"="Edit Tree Items.Set Tag", "Short name (localized)"="Edit Tree Items.Set Tag", "Long name (localized)"="Edit Tree Items:Set Tag"}, "Method Flags"={"IsDeprecated"=FALSE, "IsPrivate"=FALSE, "IsScripting"=FALSE, "IsNotInRun-Time"=FALSE}, "Divider"=FALSE}, {"Class Info"={"Unique ID string"="66", "Parent ID string"="6", "Class Name (unlocalized)"="TreeControl", "Class Name (localized)"="TreeControl"}, "Method Info"={"Unique ID string"="756a380f", "Data name"="Custom 
